vi "Meas Main.vi"(8 "error in":errorcluster, 11 "meas in":variant) -> (0 "error out":errorcluster, 3 "meas out":variant)   [LabVIEW 2013]
doc: "Main measurement VI.\nInitializes instruments, excecutes meas. loop, closes instruments."
uses:
  meas session.ctl
  Meas Sweep Config.ctl
  Meas Freq Info.ctl
  meas_swp_mode.ctl
  meas_sweep_flist_mode.ctl
  bridge/Bridge Session.ctl
  bridge/Bridge Type.ctl
  drivers/TWM client/TWM Session.ctl
  drivers/TWM client/TWM parameters.ctl
  source/Source Session.ctl
  source/Source Type.ctl
  drivers/AFG3101C/AFG3101C Session.ctl
  varilib/SGUI Assign Multiple Strings With Tags By Label.vi
  varilib/varilib.lvlib
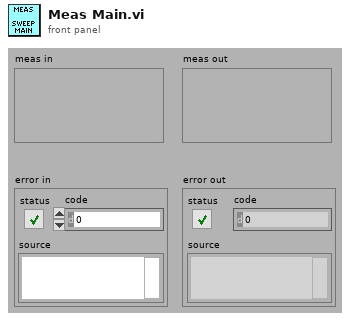
[diagram p1: front panel]
types:
  T1 = typedef "meas session.ctl" = cluster{"swp cfg":T2, "bridge":T6, "src":T10, "results":refnum<vi>}
  T2 = typedef "Meas Sweep Config.ctl" = cluster{"N":i32, "R":i32, "f list":T3[], "smpl delay":dbl, "set delay":dbl, "set delay np":dbl, "meas root":path, "meas name":string, "meas a-index":bool, "rnd sweep":bool, "mode":T4, "swp mode":T5}
  T3 = typedef "Meas Freq Info.ctl" = cluster{"f [Hz]":dbl, "periods":dbl, "f/fs":dbl, "time [s]":dbl, "fs [Hz]":dbl, "N":i32, "level":dbl, "bias":dbl}
  T4 = typedef "meas_swp_mode.ctl" = enum16{"Frequency", "Level", "Bias"}
  T5 = typedef "meas_sweep_flist_mode.ctl" = enum16{"Linear", "Log10"}
  T6 = typedef "Bridge Session.ctl" = cluster{"type":T7, "TWM":T8, "last f":dbl}
  T7 = typedef "Bridge Type.ctl" = enum16{"TWM client", "dummy"}
  T8 = typedef "TWM Session.ctl" = cluster{"pipe name":string, "parameters":T9[], "handle":i32, "fixed aper [s]":dbl}
  T9 = typedef "TWM parameters.ctl" = cluster{"name":string, "value":string[]}
  T10 = typedef "Source Session.ctl" = cluster{"type":T11, "afg":T12}
  T11 = typedef "Source Type.ctl" = enum16{"Tektronix AFG3101C", "dummy"}
  T12 = typedef "AFG3101C Session.ctl" = cluster{"VISA":refnum<visa-resource-name>, "const":dbl, "gen DC":bool}
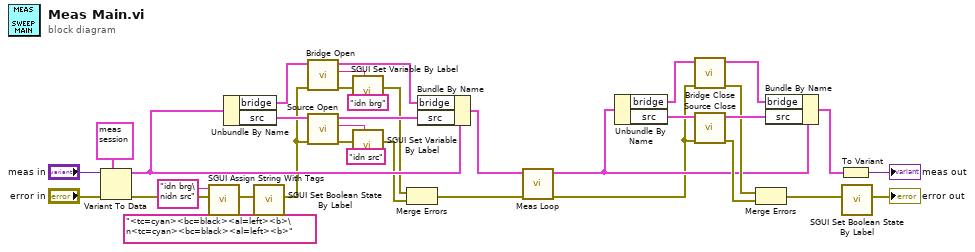
[diagram p0: block diagram]
diagram:
  n1 = Variant To Data(error in="error in", type=T1 {"swp cfg"={"N"=0, "R"=0, "f list"=[], "smpl delay"=0.0, "set delay"=0.0, "set delay np"=0.0, "meas root"=path "", "meas name"="", "meas a-index"=FALSE, "rnd sweep"=FALSE, "mode"=enum."Frequency", "swp mode"=enum."Linear"}, "bridge"={"type"=enum."TWM client", "TWM"={"pipe name"="", "parameters"=[], "handle"=0, "fixed aper [s]"=0.0}, "last f"=0.0}, "src"={"type"=enum."Tektronix AFG3101C", "afg"={"VISA"="", "const"=0.0, "gen DC"=FALSE}}, "results"=refnum} ("meas session"), Variant="meas in") -> (data=w25:T1, error out=w2:errorcluster)
  n2 = call-poly "SGUI Assign String With Tags.vi"("error in"=w2, "label(s) (empty)"="idn brg\nidn src" ("control label (none)"), "string (empty)"="<tc=cyan><bc=black><al=left><b>\n<tc=cyan><bc=black><al=left><b>") -> ("error out"=w1:errorcluster)  [unwired: 7 in, 1 out]
  n3 = Unbundle By Name(w25) -> ("bridge"=w30:T6, "src"=w31:T10)
  n4 = call "SGUI Set Boolean State By Label.vi"("error in"=w1) -> ("error out"=w14:errorcluster)  [unwired: 9 in, 1 out]
  n5 = call "Bridge Open.vi"("error in"=w14, "bridge in"=w30) -> ("error out"=w12:errorcluster, "idn string"=w10:string, "bridge out"=w26:T6)  [unwired: 7 in]
  n6 = call "Source Open.vi"("error in"=w14, "src in"=w31) -> ("error out"=w8:errorcluster, "idn string"=w6:string, "src out"=w27:T10)  [unwired: 7 in]
  n7 = call "SGUI Set Variable By Label.vi"("value (none)"=w10, "error in"=w12, "control label (none)"="idn brg") -> ("error out"=w11:errorcluster)  [unwired: 7 in, 1 out]
  n8 = call "SGUI Set Variable By Label.vi"("value (none)"=w6, "error in"=w8, "control label (none)"="idn src") -> ("error out"=w7:errorcluster)  [unwired: 7 in, 1 out]
  n9 = Merge Errors(w11, w7) -> (w13:errorcluster)
  n10 = Bundle By Name(cluster=w25, "bridge"=w26, "src"=w27) -> (w19:T1)
  n11 = call "Meas Loop.vi"("error in"=w13, "meas in"=w19) -> ("error out"=w17:errorcluster, "meas out"=w18:T1)  [unwired: 8 in]
  n12 = Unbundle By Name(w18) -> ("bridge"=w28:T6, "src"=w29:T10)
  n13 = call "Bridge Close.vi"("error in"=w17, "bridge in"=w28) -> ("error out"=w21:errorcluster, "bridge out"=w23:T6)  [unwired: 8 in]
  n14 = call "Source Close.vi"("error in"=w17, "src in"=w29) -> ("error out"=w20:errorcluster, "src out"=w24:T10)  [unwired: 8 in]
  n15 = Merge Errors(w21, w20) -> (w16:errorcluster)
  n16 = Bundle By Name(cluster=w18, "bridge"=w23, "src"=w24) -> (w22:T1)
  n17 = To Variant(anything=w22) -> (Variant=→"meas out":variant)
  n18 = call "SGUI Set Boolean State By Label.vi"("error in"=w16) -> ("error out"=→"error out":errorcluster)  [unwired: 9 in, 1 out]
